vi "Decorate Base.vi"(10 "Actor To Decorate Base":refnum<class "Actor.lvclass">) -> (2 "Decorated Base Actor":refnum<class "Actor.lvclass">)   [LabVIEW 2025, in "jettl.lvlib" / "Actor.lvlib"]
uses:
  Actor.lvlib
  Base Actor/Base Actor.lvclass
  Actor/Actor.lvclass
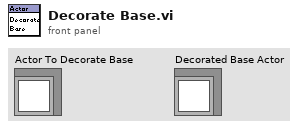
[diagram p1: front panel]
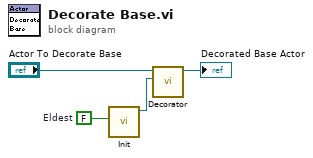
[diagram p0: block diagram]
diagram:
  w1 = FALSE  # Eldest
  n1 = call "Init.vi"("Eldest"=w1) -> ("Base Actor out"=w4:refnum<class "Base Actor.lvclass">)  [unwired: 10 in]
  n2 = call-dynamic "Decorator.vi"("Actor"=w4, "Actor in"="Actor To Decorate Base") -> ("Actor out"=→"Decorated Base Actor":refnum<class "Actor.lvclass">)  [unwired: 9 in]
